vi "Read Value with Default.vi"(6 "Gantry in":refnum<class "Gantry.lvclass">, 8 "error in (no error)":errorcluster, 9 "Default":string, 10 "String in":string, 11 "gScript Interpreter in":refnum<class "gScript Interpreter.lvclass">) -> (0 "error out":errorcluster, 2 "Memory Cell":T1, 3 "gScript Interpreter out":refnum<class "gScript Interpreter.lvclass">, 4 "Gantry out":refnum<class "Gantry.lvclass">)   [LabVIEW 2024, in "gScript Interpreter.lvclass"]
uses:
  gScript Interpreter.lvclass
  Type Definitions/Memory Cell.ctl
  Type Definitions/Memory Cell Type Enum.ctl
  Shared Components/Gantry Class/Gantry.lvclass
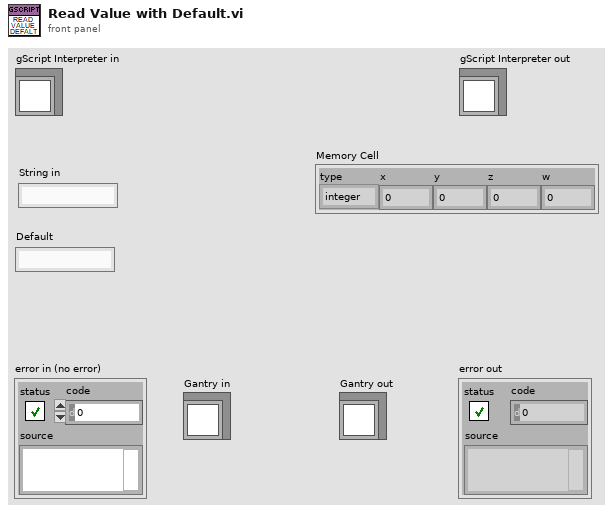
[diagram p1: front panel]
types:
  T1 = typedef "Memory Cell.ctl" = cluster{"type":T2, "x":dbl, "y":dbl, "z":dbl, "w":dbl}
  T2 = typedef "Memory Cell Type Enum.ctl" = enum16{"integer", "float", "vector", "rotation"}
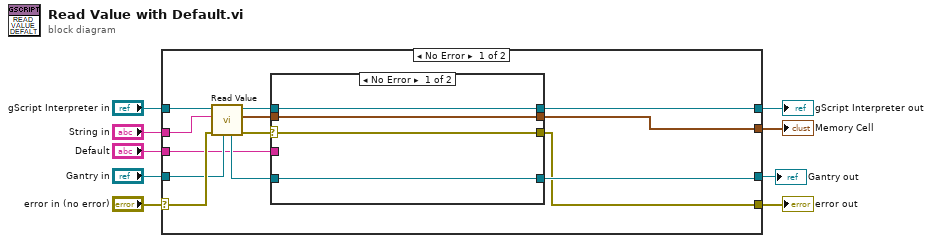
[diagram p0: block diagram]
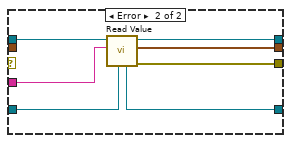
[diagram p2: hidden frame]
diagram:
  n1 = case shown="No Error" "error in (no error)" {
    selector: "error in (no error)" -> [w21 w36]
    tunnel: [w10 w36] -> w8
    tunnel: [w15 w35] -> w6
    tunnel: "gScript Interpreter in" -> [w22 w35]
    tunnel: "String in" -> [w20 _]
    tunnel: "Default" -> [w11 _]
    tunnel: "Gantry in" -> [w16 w34]
    tunnel: [w14 _] -> w2
    tunnel: [w12 w34] -> w1
    frame No Error {
      n2 = call-dynamic "Read Value.vi"("Gantry in"=w16, "error in (no error)"=w21, "String in"=w20, "gScript Interpreter in"=w22) -> ("error out"=w19:errorcluster, "Memory Cell"=w17:T1, "gScript Interpreter out"=w18:refnum<class "gScript Interpreter.lvclass">, "Gantry out"=w13:refnum<class "Gantry.lvclass">)  [unwired: 4 in]
      n3 = case shown="No Error" w19 {
        selector: w19 -> [w23 _]
        tunnel: w18 -> [w26 w33]
        tunnel: w17 -> [w25 _]
        tunnel: [w26 w32] -> w15
        tunnel: [w25 w31] -> w14
        tunnel: w13 -> [w24 w29]
        tunnel: [w24 w28] -> w12
        tunnel: w11 -> [_ w30]
        tunnel: [w23 w27] -> w10
        frame No Error {
        }
        frame Error {
          n4 = call-dynamic "Read Value.vi"("Gantry in"=w29, "String in"=w30, "gScript Interpreter in"=w33) -> ("error out"=w27:errorcluster, "Memory Cell"=w31:T1, "gScript Interpreter out"=w32:refnum<class "gScript Interpreter.lvclass">, "Gantry out"=w28:refnum<class "Gantry.lvclass">)  [unwired: 5 in]
        }
      }
    }
    frame Error {
    }
  }
  "error out" <- w8
  "gScript Interpreter out" <- w6
  "Memory Cell" <- w2
  "Gantry out" <- w1
